vi "Userdefined Symbols Array AE.vi"(8 "错误输入":errorcluster, 10 "Image In":T1[](array[typedef]), 11 "Listbox Ref":refnum<vi>) -> (0 "错误输出":errorcluster, 2 "Image Out":T1[](array[typedef]), 3 "Dup Listbox Ref":refnum<vi>)   [LabVIEW 2012, in "Listbox Tool.lvlib"]
uses:
  Listbox Tool.lvlib
  <vilib>/picture/picture.llb/imagedata.ctl
panel:
  in  "Mode":enum16{"Set", "Get", "Restore"}(ring)
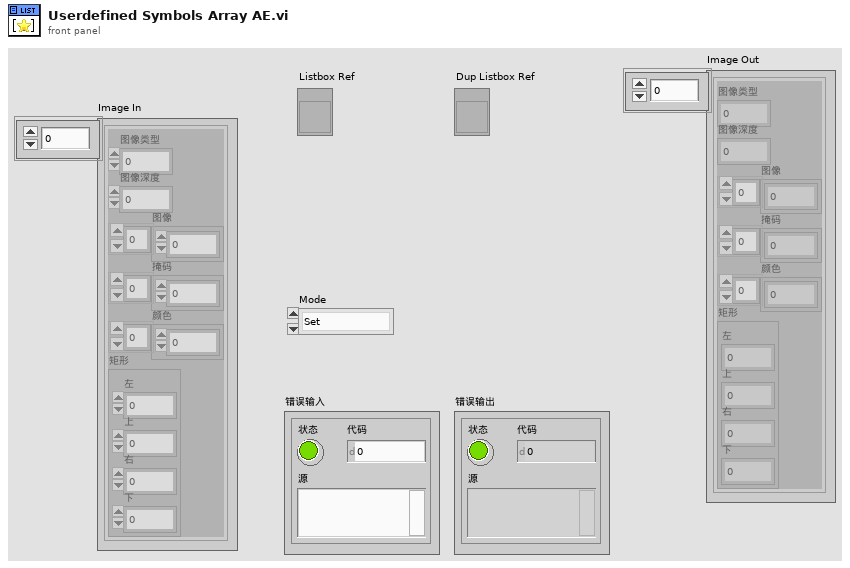
[diagram p1: front panel]
types:
  T1 = typedef "imagedata.ctl" = cluster{"image type":i32, "image depth":i32, "image":u8[], "mask":u8[], "colors":u32[], "Rectangle":cluster{"left":i16, "top":i16, "right":i16, "bottom":i16}}
  T2 = cluster{"image type":i32, "image depth":i32, "image":u8[], "mask":u8[], "colors":u32[], "Rectangle":cluster{"left":i16, "top":i16, "right":i16, "bottom":i16}}[]
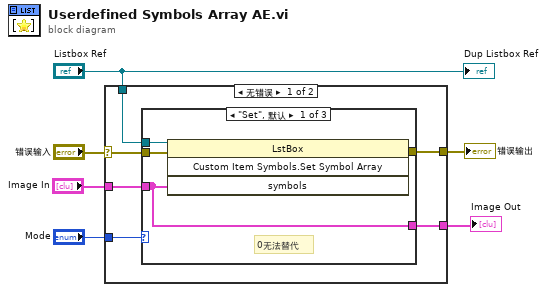
[diagram p0: block diagram]
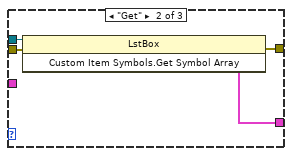
[diagram p2: hidden frame]
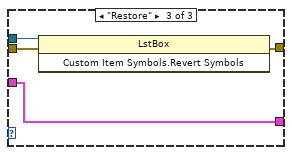
[diagram p3: hidden frame]
diagram:
  n1 = case shown="无错误" "错误输入" {
    selector: "错误输入" -> [w11 w26]
    tunnel: [w10 w26] -> w5
    tunnel: "Listbox Ref" -> [w12 _]
    tunnel: "Mode" -> [w9 _]
    tunnel: "Image In" -> [w8 w25]
    tunnel: [w7 w25] -> w1
    frame No Error {
      n2 = case shown="\"Set\", 默认" w9 {
        tunnel: w12 -> [w15 w20 w23]
        tunnel: w11 -> [w16 w19 w24]
        tunnel: [w14 w18 w22] -> w10
        tunnel: [w13 w17 w21] -> w7
        tunnel: w8 -> [w13 _ w21]
        frame "Set", Default {
          # "0无法替代"
          n3 = invoke class="LstBox" method="Custom Item Symbols.Set Symbol Array"(reference=w15, error in=w16, "symbols"=w13) -> (error out=w14:errorcluster)  [unwired: 1 in, 3 out]
        }
        frame "Get" {
          n4 = invoke class="LstBox" method="Custom Item Symbols.Get Symbol Array"(reference=w20, error in=w19) -> (error out=w18:errorcluster, "Custom Item Symbols:Get Symbol Array"=w17:T2)  [unwired: 1 in, 1 out]
        }
        frame "Restore" {
          n5 = invoke class="LstBox" method="Custom Item Symbols.Revert Symbols"(reference=w23, error in=w24) -> (error out=w22:errorcluster)  [unwired: 1 in, 2 out]
        }
      }
    }
    frame Error {
    }
  }
  "错误输出" <- w5
  "Image Out" <- w1
  "Dup Listbox Ref" <- "Listbox Ref"
